vi "CheckROIEdges (SubVI).vi"(6 "image size":i32[](array[numeric])=[1200, 1200], 7 "Bead Array":i32[][](array[numeric])=[[0, 0], [10, 0], [30, 10], [100, 100], [1000, 900], [1100, 500], [1200, 1300]], 9 "error out 2":errorcluster, 11 "front panel settings.Calibs.ROI(pix)":i32=120) -> (1 "error out":errorcluster, 5 "Bead Array adapted":i32[][](array[numeric]))   [LabVIEW 2011]
panel:
  out "Array":bool[][](array[boolean])
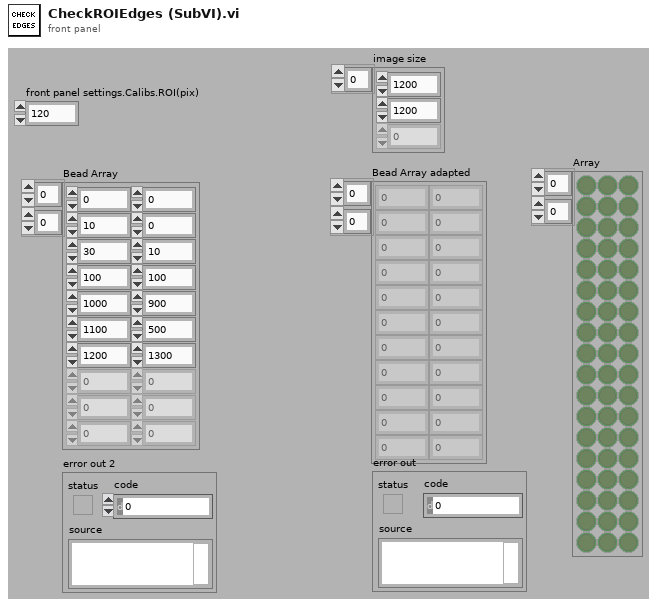
[diagram p1: front panel]
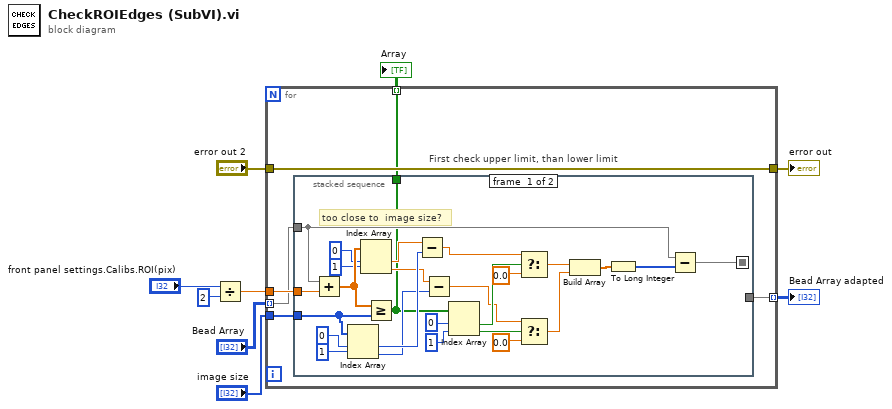
[diagram p0: block diagram]
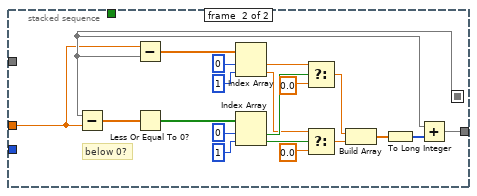
[diagram p2: hidden frame]
diagram:
  n1 = Divide(x="front panel settings.Calibs.ROI(pix)", y=2) -> (x/y=w3:dbl)
  n2 = for {
    tunnel: "Bead Array" -> [w12] mode=indexing
    tunnel: [w15] -> w5
    tunnel: "error out 2" -> [w15]
    tunnel: "image size" -> [w13]
    tunnel: w3 -> [w14]
    tunnel: [w11] -> w2 mode=indexing
    tunnel: [w10] -> w1 mode=indexing
    n3 = stacked-sequence "First check upper limit, than lower limit" {
      seq-local: [w31 _] -> [_ w46]
      tunnel: w14 -> [w30 w42]
      tunnel: w13 -> [w23 _]
      tunnel: w12 -> [w33 _]
      tunnel: [_ w50] -> w11
      tunnel: [w16 _] -> w10
      frame #0 {
        # "too close to  image size?"
        n4 = Add(x=w33, y=w30) -> (x+y=w28:dbl[])
        n5 = Index Array(array=w23, index #1=0 ("index"), index #2=1 ("index")) -> (element #1=w22:i32, element #2=w17:i32)
        n6 = Index Array(array=w28, index #1=0 ("index"), index #2=1 ("index")) -> (element #1=w21:dbl, element #2=w18:dbl)
        n7 = Greater Or Equal?(x=w28, y=w23) -> (x >= y?=w16:bool[])
        n8 = Subtract(x=w21, y=w22) -> (x-y=w20:dbl)
        n9 = Subtract(x=w18, y=w17) -> (x-y=w19:dbl)
        n10 = Index Array(array=w16, index #1=0 ("index"), index #2=1 ("index")) -> (element #1=w39:bool, element #2=w38:bool)
        n11 = Select(t=w20, s=w39, f=0.0) -> (s? t:f=w35:dbl)
        n12 = Select(t=w19, s=w38, f=0.0) -> (s? t:f=w34:dbl)
        n13 = Build Array(w35, w34) -> (w32:dbl[])
        n14 = To Long Integer(number=w32) -> (32bit integer=w29:i32[])
        n15 = Subtract(x=w33, y=w29) -> (x-y=w31:i32[])
      }
      frame #1 {
        # "below 0?"
        n16 = Subtract(x=w46, y=w42) -> (x-y=w49:dbl[])
        n17 = Subtract(x=w42, y=w46) -> (x-y=w45:dbl[])
        n18 = Less Or Equal To 0?(x=w49) -> (x <= 0?=w61:bool[])
        n19 = Index Array(array=w45, index #1=0 ("index"), index #2=1 ("index")) -> (element #1=w44:dbl, element #2=w43:dbl)
        n20 = Index Array(array=w61, index #1=0 ("index"), index #2=1 ("index")) -> (element #1=w58:bool, element #2=w57:bool)
        n21 = Select(t=w44, s=w58, f=0.0) -> (s? t:f=w54:dbl)
        n22 = Select(t=w43, s=w57, f=0.0) -> (s? t:f=w53:dbl)
        n23 = Build Array(w54, w53) -> (w52:dbl[])
        n24 = To Long Integer(number=w52) -> (32bit integer=w51:i32[])
        n25 = Add(x=w46, y=w51) -> (x+y=w50:i32[])
      }
    }
  }
  "Bead Array adapted" <- w2
  "error out" <- w5
  "Array" <- w1
